vi "ExitGui.vi"(11 "Message":string) -> (2 "ok":bool, 3 "ExitAction":T1=enum."Shut Down PC")   [LabVIEW 2016]
uses:
  tools/Windows/Windows.ExitAction.ctl
  ExitGui.Action.ctl
  tools/Translator/Translator.Global.vi
  Global/ApplicationGlobal.vi
panel:
  out "_loop":i32(ring)=4
  in  "ExitOption":u16(ring)=3
  in  "CancelButton":bool
  in  "OKButton":bool
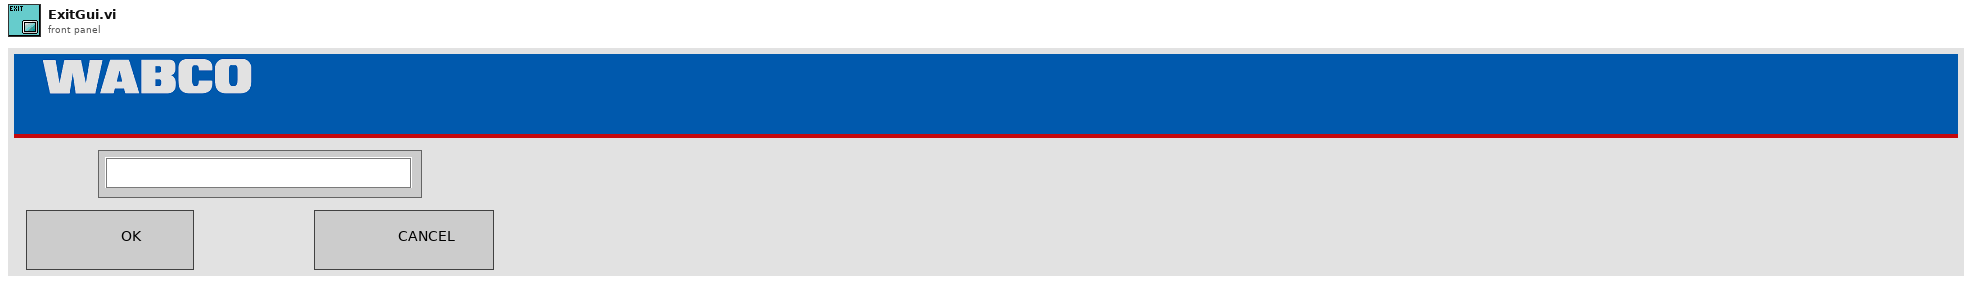
[diagram p1: front panel]
types:
  T1 = typedef "Windows.ExitAction.ctl" = enum16{"Log off from PC", "Shut Down PC", "Reboot PC", "Close Program"}
  T2 = typedef "ExitGui.Action.ctl" = enum32{"idle", "constructor", "destructor", "--- ExitGUI ---"}
  T3 = enum32{"Invalid", "Default", "Floating", "Floating/Auto-Hide", "Modal"}
  T4 = typedef "FestoCPX.Station.ButtonsState.ctl" = cluster{"Start":bool, "Stop":bool, "Control":bool}
  T5 = typedef "LVPositionTypeDef.ctl" = cluster{"Left":i32, "Top":i32}
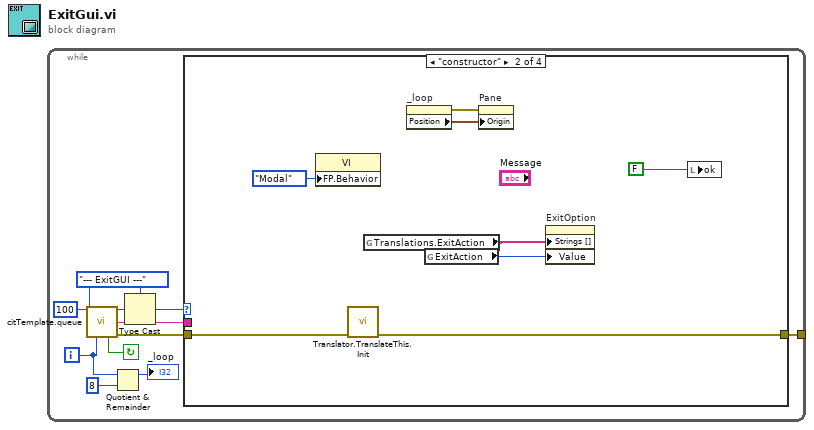
[diagram p0: block diagram]
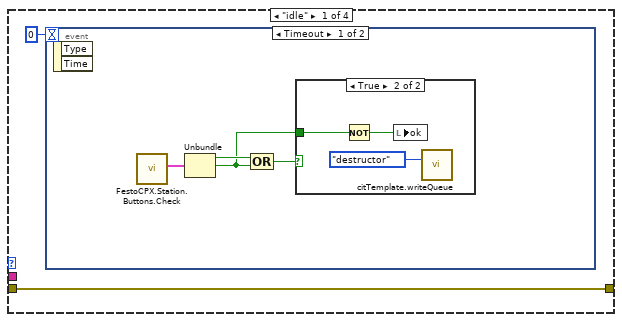
[diagram p2: hidden frame]
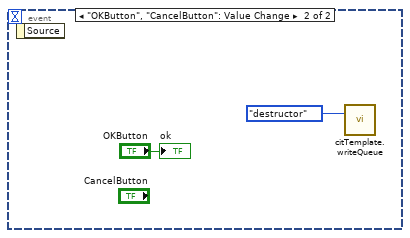
[diagram p4: hidden frame]
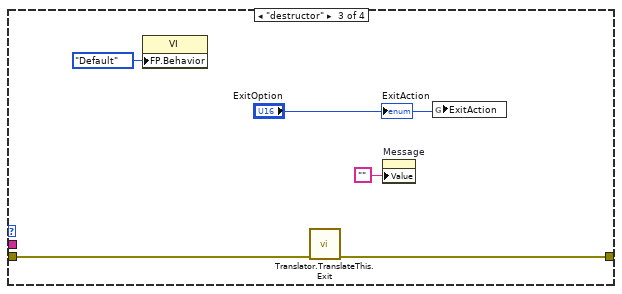
[diagram p5: hidden frame]
diagram:
  n1 = while {
    tunnel: [w1] -> _
    i -> [w2]
    stop <- w11 continue-if-true
    w5 = ExitGui.Action."--- ExitGUI ---" ("Action")
    n2 = call "citTemplate.queue.vi"("ms timeout (250 ms)"=100, "event enum"=w5, "iteration (-1)"=w2) -> ("event out"=w9:u32, "(flatten) data out"=w6:string, "continue"=w11:bool, "error out"=w7:errorcluster)  [unwired: 2 in, 7 out]
    n3 = Quotient & Remainder(x=w2, y=8) -> (x-y*floor(x/y)=→"_loop":i32)  [unwired: 1 out]
    n4 = Type Cast(type=w5, x=w9) -> (*(type *) &x=w8:T2)
    n5 = case shown="\"constructor\"" w8 {
      tunnel: w7 -> [w12 w25 w33 w36]
      tunnel: w6 -> [_ _ _ _]
      tunnel: [w12 w24 w32 w36] -> w1
      frame "idle" {
        n6 = event shown="[0] Timeout" {
          selector: _ -> [_ _]
          dyn-events: _ -> [_ _]
          timeout: 0 -> [_ _]
          event Timeout {
            n7 = event-data() -> ()  [unwired: 3 out]
            n8 = call "FestoCPX.Station.Buttons.Check.vi"() -> ("Buttons.State"=w17:T4)  [unwired: 10 in, 1 out]
            n9 = Unbundle(w17) -> ("Start"=w16:bool, "Stop"=w14:bool)  [unwired: 1 out]
            n10 = Compound Arithmetic op=OR(w16, w14) -> (w15:bool)
            n11 = case shown="True" w15 {
              tunnel: w14 -> [_ w20]
              frame False {
              }
              frame True {
                n12 = Not(x=w20) -> (.not. x?=w19:bool)
                n13 = local write "ok"(w19) -> ()
                n14 = call "citTemplate.writeQueue.vi"("event in (if not connected:all statemachine with data event)"=ExitGui.Action."destructor" ("Action")) -> ()  [unwired: 14 in, 1 out]
              }
            }
          }
          event "OKButton", "CancelButton": Value Change {
            n15 = event-data() -> ()  [unwired: 2 out]
            n16 = call "citTemplate.writeQueue.vi"("event in (if not connected:all statemachine with data event)"=ExitGui.Action."destructor" ("Action")) -> ()  [unwired: 14 in, 1 out]
            "ok" <- "OKButton"
          }
        }
      }
      frame "constructor" {
        n17 = property class="VI"("FP.Behavior"=T3."Modal" ("Front Panel Window:Behavior")) -> ()  [unwired: 2 in, 2 out]
        n18 = call "Translator.TranslateThis.Init.vi"("error in"=w25) -> ("error out"=w24:errorcluster)  [unwired: 10 in]
        n19 = global read "Translator.Global.vi" "Translations.ExitAction"() -> (w27:string[])
        n20 = property on="_loop" class="Ring (strict)"() -> (error out=w28:errorcluster, "Position"=w29:T5)  [unwired: 2 in, 1 out]
        n21 = global read "ApplicationGlobal.vi" "ExitAction"() -> (w26:T1)
        n22 = property on="Pane" class="Pane"(error in=w28, "Origin"=w29) -> ()  [unwired: 1 in, 2 out]
        n23 = property on="ExitOption" class="Ring (strict)"("Strings []"=w27, "Value"=w26) -> ()  [unwired: 2 in, 2 out]
        n24 = local write "ok"(FALSE ("_b_ok")) -> ()
      }
      frame "destructor" {
        n25 = property class="VI"("FP.Behavior"=T3."Default" ("Front Panel Window:Behavior")) -> ()  [unwired: 2 in, 2 out]
        n26 = call "Translator.TranslateThis.Exit.vi"("error in"=w33) -> ("error out"=w32:errorcluster)  [unwired: 10 in]
        n27 = property on="Message" class="Str"("Value"="") -> ()  [unwired: 2 in, 2 out]
        n28 = global write "ApplicationGlobal.vi" "ExitAction"("ExitOption") -> ()
        "ExitAction" <- "ExitOption"
      }
      frame "--- ExitGUI ---" {
      }
    }
  }
